vi "SubVI to Code.vi"(10 "C code in":string, 11 "reference":refnum<vi>) -> (2 "C code":string, 3 "SubVI terminals info":T1)   [LabVIEW 2014]
panel:
  in  "error in":errorcluster
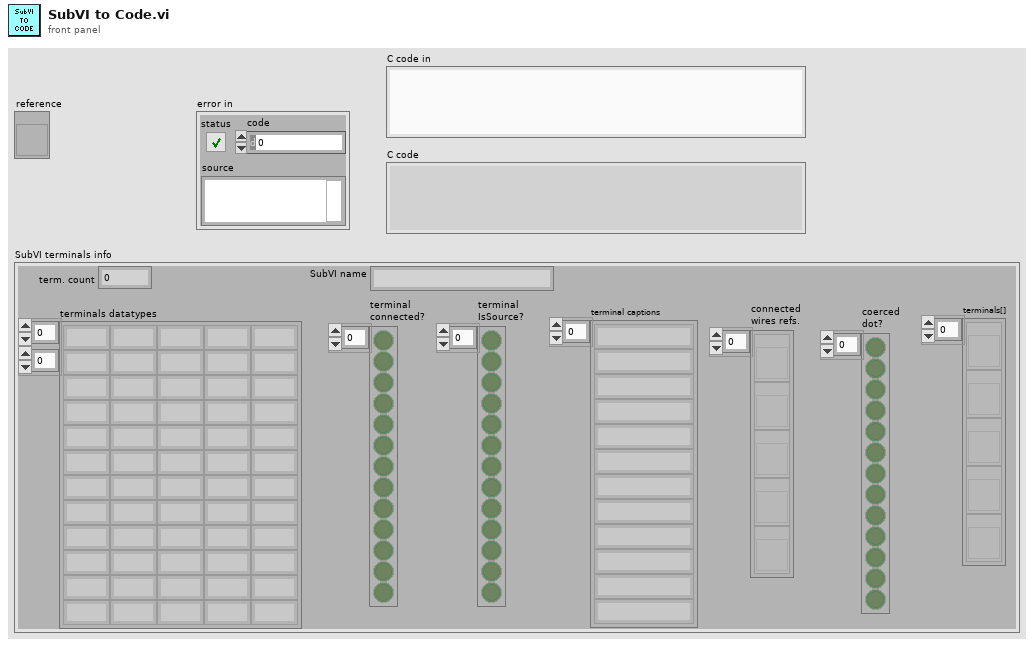
[diagram p1: front panel]
types:
  T1 = cluster{"terminals datatypes":string[][], "terminal\nconnected?":bool[], "terminal captions":string[], "term. count":i32, "terminal\nIsSource?":bool[], "SubVI name":string, "connected\nwires refs.":refnum<vi>[], "coerced\ndot?":bool[], "terminals[]":refnum<vi>[]}
  T2 = cluster{"terminals datatypes":string[][], "terminal\nconnected?":bool[], "terminal captions":string[], "term. count":i32, "terminal\nIsSource?":bool[], "SubVI name":string, "connected\nwires refs.":refnum<vi>[], "coerced dot?":bool[], "terminals[]":refnum<vi>[]}
  T3 = cluster{"wire labels":string[], "wire terminals datatypes":string[][]}
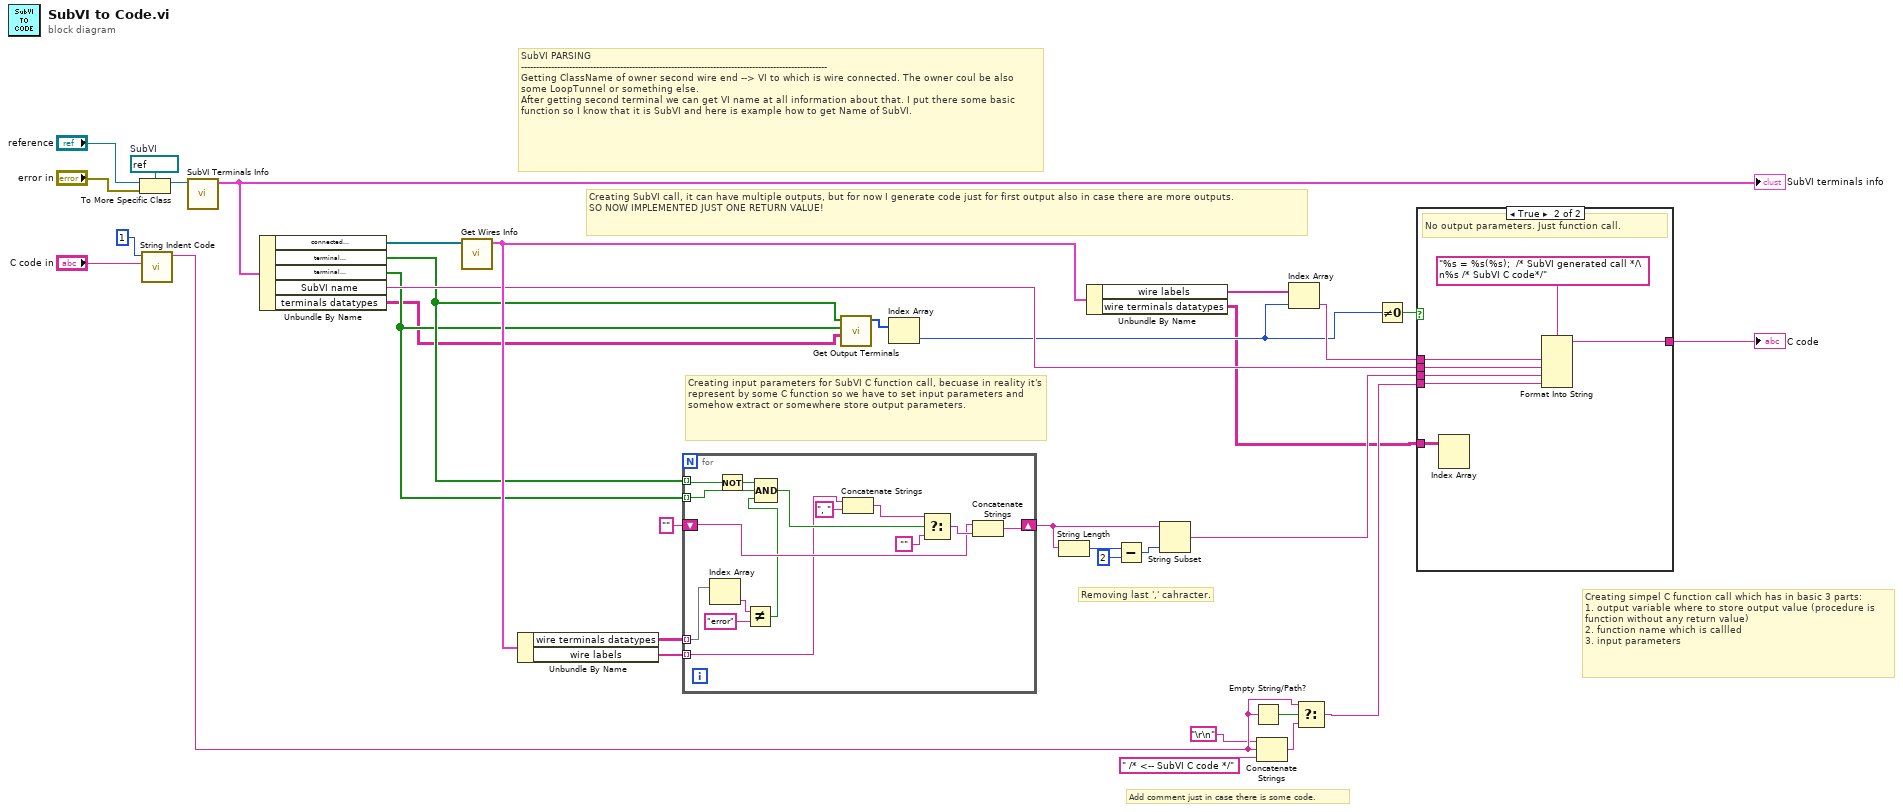
[diagram p0: block diagram]
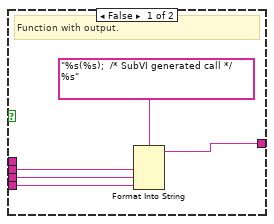
[diagram p2: hidden frame]
diagram:
  w21 = refnum<vi> refnum  # SubVI
  # "Add comment just in case there is some code."
  # "Creating SubVI call, it can have multiple outputs, but for now I generate code just for first output also in case there are more outputs.\nSO NOW IMPLEMENTED JUST ONE RETURN VALUE!"
  # "Creating simpel C function call which has in basic 3 parts:\n1. output variable where to store output value (procedure is function without any return value)\n2. function name which is callled\n3. input parameters"
  # "Removing last ',' cahracter."
  # "Creating input parameters for SubVI C function call, becuase in reality it's represent by some C function so we have to set input parameters and somehow extract or somewhere store output parameters."
  # "SubVI PARSING\n------------------------------------------------------------------------------------------------------\nGetting ClassName of owner second wire end --> VI to which is wire connected. The owner coul be also some LoopTunnel or something else.\nAfter getting second terminal we can get VI name at all information about that. I put there some basic function so I know that it is SubVI and here is example how to get Name of SubVI."
  n1 = To More Specific Class(target class=w21, reference="reference", error in="error in") -> (specific class reference=w22:refnum<vi>)  [unwired: 1 out]
  n2 = call "String Indent Code.vi"("complete code"="C code in", "actual nested level"=1) -> ("indented code"=w4:string)  [unwired: 9 in]
  n3 = call "SubVI Terminals Info.vi"("SubVI ref"=w22) -> ("output cluster"=w24:T2)  [unwired: 9 in, 1 out]
  "SubVI terminals info" <- w24
  n4 = Unbundle By Name(w24) -> ("connected\nwires refs."=w23:refnum<vi>[], "terminal\nIsSource?"=w17:bool[], "terminal\nconnected?"=w16:bool[], "SubVI name"=w28:string, "terminals datatypes"=w15:string[][])
  n5 = call "Get Wires Info.vi"("connected\nwires refs."=w23) -> ("output cluster 2"=w30:T3)  [unwired: 10 in]
  n6 = Unbundle By Name(w30) -> ("wire terminals datatypes"=w18:string[][], "wire labels"=w31:string[])
  n7 = for {
    tunnel: w17 -> [w49] mode=indexing
    tunnel: w16 -> [w48] mode=indexing
    shift-right: [w42] -> w25
    shift-left: "" -> [w43]
    tunnel: w31 -> [w38] mode=indexing
    tunnel: w18 -> [w36] mode=indexing
    n8 = Index Array(array=w36) -> (element=w35:string)  [unwired: 1 in]
    n9 = Not(x=w49) -> (.not. x?=w45:bool)
    n10 = Not Equal?(x=w35, y="error") -> (x != y?=w37:bool)
    n11 = Compound Arithmetic op=AND(w45, w48, w37) -> (w47:bool)
    n12 = Concatenate Strings(w38, ", " ("string")) -> (w40:string)
    n13 = Select(t=w40, s=w47, f="") -> (s? t:f=w44:string)
    n14 = Concatenate Strings(w43, w44) -> (w42:string)
  }
  n15 = call "Get Output Terminals.vi"("terminals datatypes"=w15, "isSource?"=w16, "isConnected?"=w17) -> ("output terminals indexes"=w14:i32[])  [unwired: 8 in]
  n16 = Index Array(array=w14) -> (element=w10:i32)  [unwired: 1 in]
  n17 = String Length(string=w25) -> (length=w33:i32)
  n18 = Unbundle By Name(w30) -> ("wire labels"=w27:string[], "wire terminals datatypes"=w1:string[][])
  n19 = Subtract(x=w33, y=2) -> (x-y=w32:i32)
  n20 = String Subset(string=w25, length (rest)=w32) -> (substring=w13:string)  [unwired: 1 in]
  n21 = Empty String/Path?(string/path=w4) -> (empty?=w7:bool)
  n22 = Concatenate Strings("\r\n", w4, " /* <-- SubVI C code */" ("string")) -> (w6:string)
  n23 = Index Array(array=w27, index=w10) -> (element=w12:string)
  n24 = Select(t=w4, s=w7, f=w6) -> (s? t:f=w5:string)
  n25 = Not Equal To 0?(x=w10) -> (x != 0?=w11:bool)
  n26 = case shown="True" w11 {
    tunnel: [w54 w61] -> w29
    tunnel: w28 -> [w53 w60]
    tunnel: w12 -> [_ w59]
    tunnel: w13 -> [w51 w57]
    tunnel: w5 -> [w50 w56]
    tunnel: w1 -> [_ w55]
    frame False {
      # "Function with output."
      n27 = Format Into String(format string="%s(%s);  /* SubVI generated call */ %s", w53, w51, w50) -> (resulting string=w54:string)  [unwired: 2 in, 1 out]
    }
    frame True {
      # "No output parameters. Just function call."
      n28 = Index Array(array=w55) -> ()  [unwired: 2 in, 1 out]
      n29 = Format Into String(format string="%s = %s(%s);  /* SubVI generated call */\n%s /* SubVI C code*/", w59, w60, w57, w56) -> (resulting string=w61:string)  [unwired: 2 in, 1 out]
    }
  }
  "C code" <- w29
